vi "AET_Algorithms.vi"(8 "error in":errorcluster, 11 "Image In":T5) -> (0 "error IO":errorcluster, 3 "Mesurement Value":sgl)   [LabVIEW 2019, in "Algorithm.lvclass"]
uses:
  FrameworkOverrides/Algorithm.lvclass
  <vilib>/vision/Measure.llb/Edge Polarity.ctl
  <vilib>/vision/Measure.llb/Edge Options.ctl
  <vilib>/vision/Image Controls.llb/IMAQ Image.ctl
panel:
  in  "Measurement Type":string
  in  "Zen Algo":string
  in  "Reference Edge Search Direction":u32(ring) items=["Left to Right", "Right to Left", "Top to Bottom", "Bottom to Top"]
  in  "Process":T1(ring)=enum."Get All Edges"
  in  "Edge Options":T2={"Edge Polarity"=0, "Kernel Size"=3, "Width"=3, "Minimum Edge Strength"=10.0, "Interpolation Type"=enum."Bilinear Fixed", "Data Processing Method"=enum."Average"} {"Edge Polarity" items=["All Edges", "Rising Edges", "Falling Edges"]; "Minimum Edge Strength" format="%.2f"; "Width" step=2; "Kernel Size" step=2}
  in  "ROI":T4 {"Rotation" format="%.2f"; "Left" scale=0.0..1024.0; "Right" scale=0.0..1024.0}
  in  "Step Size":u32
  in  "Calibrated Image":T5
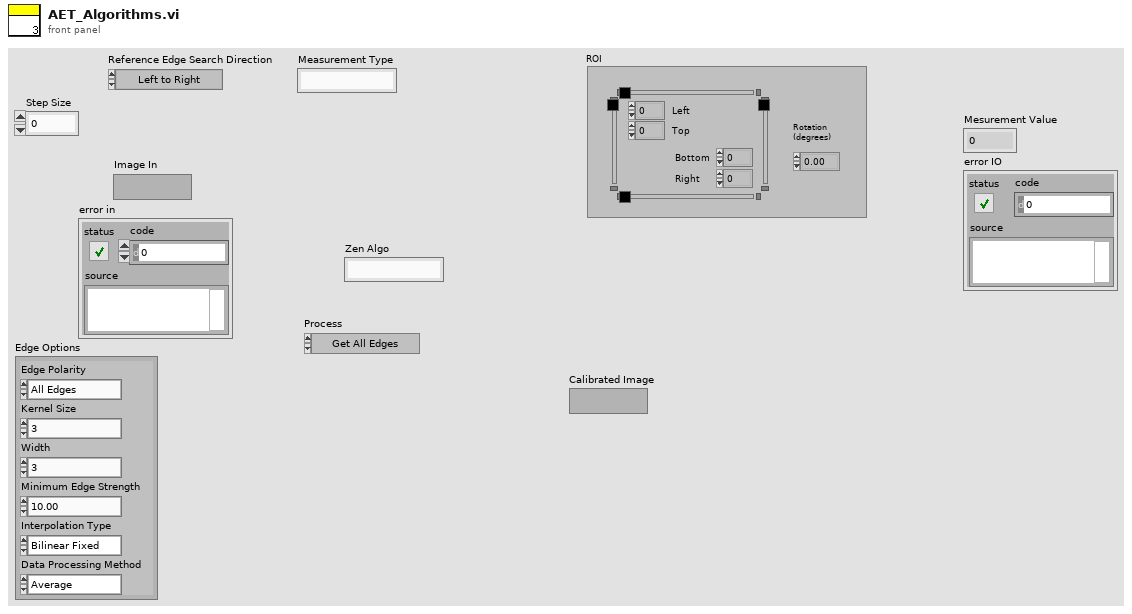
[diagram p1: front panel]
types:
  T1 = enum16{"Get First Edge", "Get First + Last Edge", "Get All Edges", "Get Best Edge"}
  T2 = typedef "Edge Options.ctl" = cluster{"Edge Polarity":T3, "Kernel Size":u32, "Width":u32, "Minimum Edge Strength":sgl, "Interpolation Type":enum32{"Zero Order", "Bilinear", "Quadratic", "Cubic", "Bilinear Fixed"}, "Data Processing Method":enum32{"Average", "Median"}}
  T3 = typedef "Edge Polarity.ctl" = u32
  T4 = typedef "IMAQ Rectangle" = cluster{"Left":i32, "Top":i32, "Right":i32, "Bottom":i32, "Rotation":dbl}
  T5 = typedef "IMAQ Image.ctl" = refnum<image>
  T6 = cluster{"Contrast":i32, "Filter width":i32, "Steepness":i32, "Subsampling Ratio":u32, "Show Search Area":bool, "Show Search Lines":bool, "Show Edges Found":bool, "Show Result":bool}
  T7 = typedef "ROI Descriptor" = cluster{"Global Rectangle":i32[], "Contours":cluster{"ID":enum32{"External", "Internal"}, "Type":u32, "Coordinates":i32[]}[]}
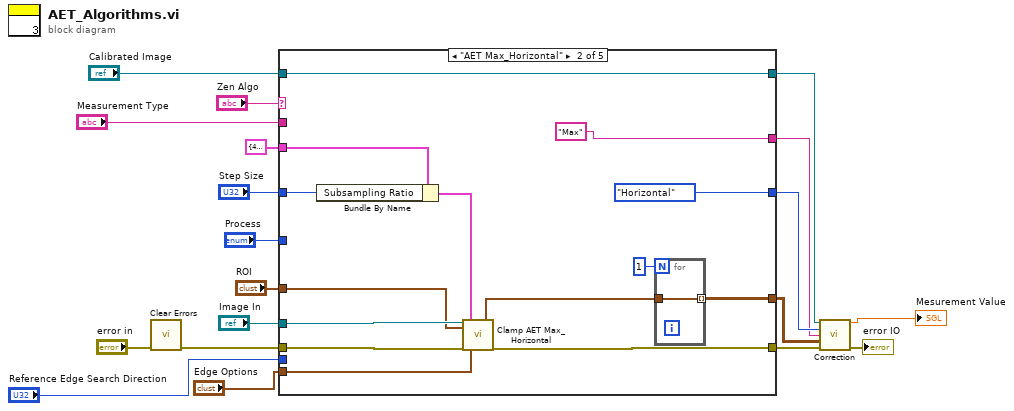
[diagram p0: block diagram]
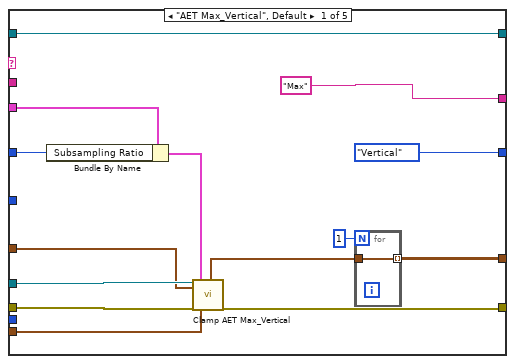
[diagram p2: hidden frame]
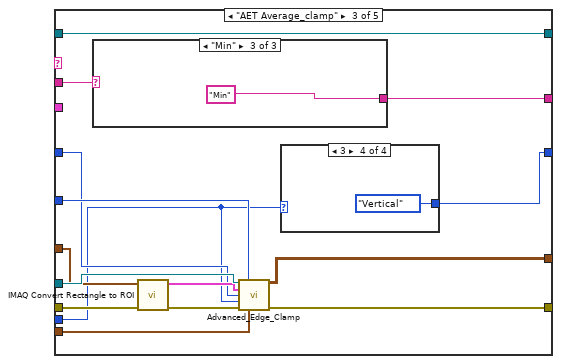
[diagram p3: hidden frame]
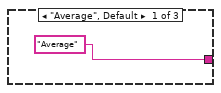
[diagram p4: hidden frame]
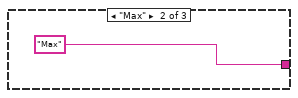
[diagram p5: hidden frame]
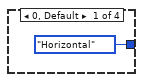
[diagram p6: hidden frame]
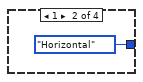
[diagram p7: hidden frame]
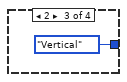
[diagram p8: hidden frame]
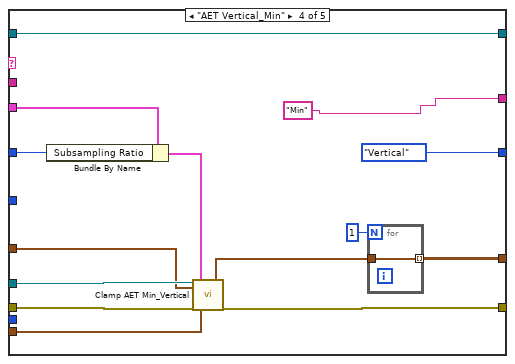
[diagram p9: hidden frame]
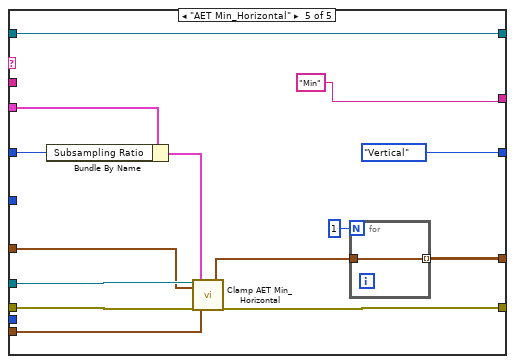
[diagram p10: hidden frame]
diagram:
  n1 = call <vilib>:"Clear Errors.vi"("error in (no error)"="error in") -> ("error out"=w11:errorcluster)  [unwired: 5 in, 1 out]
  n2 = case shown="\"AET Max_Horizontal\"" "Zen Algo" {
    tunnel: "Measurement Type" -> [_ _ w61 _ _]
    tunnel: "Image In" -> [w27 w48 w64 w85 w100]
    tunnel: "Edge Options" -> [w33 w47 w62 w81 w99]
    tunnel: [w32 w46 w60 w84 w98] -> w18
    tunnel: [w23 w38 w59 w75 w89] -> w17
    tunnel: [enum16{"Horizontal", "Vertical"}."Vertical" ("Search Direction") enum16{"Horizontal", "Vertical"}."Horizontal" ("Search Direction") w58 enum16{"Horizontal", "Vertical"}."Vertical" ("Search Direction") enum16{"Horizontal", "Vertical"}."Vertical" ("Search Direction")] -> w16
    tunnel: ["Max" "Max" w57 "Min" "Min"] -> w1
    tunnel: w11 -> [w30 w44 w56 w82 w96]
    tunnel: T6 {"Contrast"=40, "Filter width"=4, "Steepness"=2, "Subsampling Ratio"=5, "Show Search Area"=FALSE, "Show Search Lines"=FALSE, "Show Edges Found"=TRUE, "Show Result"=TRUE} ("Settings") -> [w28 w42 _ w79 w94]
    tunnel: [w26 w41 w54 w78 w93] -> w10
    tunnel: "Calibrated Image" -> [w26 w41 w54 w78 w93]
    tunnel: "Step Size" -> [w25 w40 w52 w77 w91]
    tunnel: "ROI" -> [w24 w39 w51 w76 w92]
    tunnel: "Process" -> [_ _ w53 _ _]
    tunnel: "Reference Edge Search Direction" -> [_ _ w50 _ _]
    frame "AET Max_Vertical", Default {
      n3 = Bundle By Name(cluster=w28, "Subsampling Ratio"=w25) -> (w29:T6)
      n4 = call "Clamp AET Max_Vertical.vi"("Image"=w27, "Rectangle"=w24, "error in (no error)"=w30, "Settings"=w29, "Edge Options"=w33) -> ("Edge Coordinates"=w22:cluster{"X":sgl, "Y":sgl}[], "error out"=w32:errorcluster)  [unwired: 7 in, 6 out]
      n5 = for {
        N: 1 -> [_]
        tunnel: [w34] -> w23 mode=indexing
        tunnel: w22 -> [w34]
      }
    }
    frame "AET Max_Horizontal" {
      n6 = Bundle By Name(cluster=w42, "Subsampling Ratio"=w40) -> (w43:T6)
      n7 = call "Clamp AET Max_Horizontal.vi"("Image"=w48, "Rectangle"=w39, "error in (no error)"=w44, "Settings"=w43, "Edge Options"=w47) -> ("Edge Coordinates"=w37:cluster{"X":sgl, "Y":sgl}[], "error out"=w46:errorcluster)  [unwired: 7 in, 6 out]
      n8 = for {
        N: 1 -> [_]
        tunnel: [w49] -> w38 mode=indexing
        tunnel: w37 -> [w49]
      }
    }
    frame "AET Average_clamp" {
      n9 = case shown="\"Min\"" w61 {
        tunnel: ["Average" "Max" "Min"] -> w57
        frame "Average", Default {
        }
        frame "Max" {
        }
        frame "Min" {
        }
      }
      n10 = call "IMAQ Convert Rectangle to ROI"("error in (no error)"=w56, "Rectangle"=w51) -> ("error out"=w55:errorcluster, "ROI Descriptor"=w63:T7)  [unwired: 7 in]
      n11 = call "Advanced_Edge_Clamp.vi"("Image"=w64, "Process"=w53, "ROI Descriptor"=w63, "Step Size"=w52, "Search Direction"=w50, "error in (no error)"=w55, "Edge Options"=w62) -> ("Edge Points-Array"=w59:cluster{"X":sgl, "Y":sgl}[][], "error out"=w60:errorcluster)  [unwired: 4 in, 3 out]
      n12 = case shown="3" w50 {
        tunnel: [enum16{"Horizontal", "Vertical"}."Horizontal" ("Search Direction") enum16{"Horizontal", "Vertical"}."Horizontal" ("Search Direction") enum16{"Horizontal", "Vertical"}."Vertical" ("Search Direction") enum16{"Horizontal", "Vertical"}."Vertical" ("Search Direction")] -> w58
        frame 0, Default {
        }
        frame 1 {
        }
        frame 2 {
        }
        frame 3 {
        }
      }
    }
    frame "AET Vertical_Min" {
      n13 = Bundle By Name(cluster=w79, "Subsampling Ratio"=w77) -> (w80:T6)
      n14 = call "Clamp AET Min_Vertical.vi"("Image"=w85, "Rectangle"=w76, "error in (no error)"=w82, "Settings"=w80, "Edge Options"=w81) -> ("Edge Coordinates"=w74:cluster{"X":sgl, "Y":sgl}[], "error out"=w84:errorcluster)  [unwired: 6 in, 7 out]
      n15 = for {
        N: 1 -> [_]
        tunnel: [w86] -> w75 mode=indexing
        tunnel: w74 -> [w86]
      }
    }
    frame "AET Min_Horizontal" {
      n16 = Bundle By Name(cluster=w94, "Subsampling Ratio"=w91) -> (w95:T6)
      n17 = call "Clamp AET Min_Horizontal.vi"("Image"=w100, "Rectangle"=w92, "error in (no error)"=w96, "Settings"=w95, "Edge Options"=w99) -> ("Edge Coordinates"=w90:cluster{"X":sgl, "Y":sgl}[], "error out"=w98:errorcluster)  [unwired: 6 in, 7 out]
      n18 = for {
        N: 1 -> [_]
        tunnel: w90 -> [w101]
        tunnel: [w101] -> w89 mode=indexing
      }
    }
  }
  n19 = call "Correction.vi"("Calibrated Image"=w10, "Vertical/Horizontal"=w16, "Algo Type"=w1, "appended array"=w17, "error in (no error)"=w18) -> ("Mesurement Value"=→"Mesurement Value":sgl, "error IO"=→"error IO":errorcluster)  [unwired: 8 in, 1 out]
